vi "DrawPaticle.vi"(1 "Particle Measurements (Pixels) (左引脚)":dbl[][](array[numeric]), 2 "引用句柄输入":T1) -> (0 "Paticle中心数组":cluster{"Numeric":dbl, "Numeric":dbl}[](array[cluster]))   [LabVIEW 2014]
uses:
  <vilib>/vision/Image Controls.llb/IMAQ Image.ctl
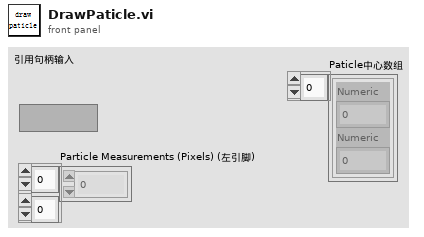
[diagram p1: front panel]
types:
  T1 = typedef "IMAQ Image.ctl" = refnum<image>
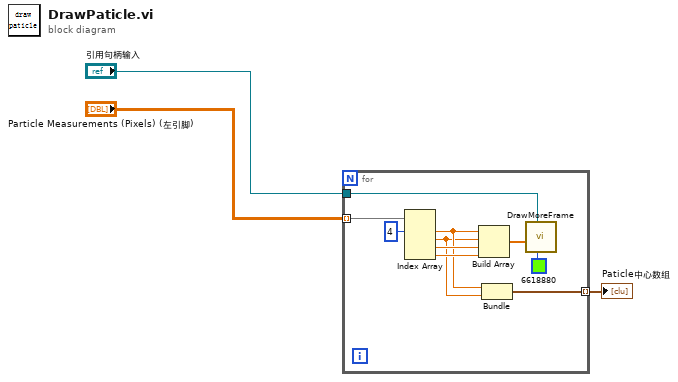
[diagram p0: block diagram]
diagram:
  n1 = for {
    tunnel: "Particle Measurements (Pixels) (左引脚)" -> [w13] mode=indexing
    tunnel: "引用句柄输入" -> [w9]
    tunnel: [w4] -> w1 mode=indexing
    n2 = Index Array(array=w13, index #1=4 ("索引")) -> (element #1=w6:dbl, element #2=w5:dbl, element #3=w12:dbl, element #4=w11:dbl)  [unwired: 3 in]
    n3 = Build Array(w6, w5, w12, w11) -> (w10:dbl[])
    n4 = Bundle("Numeric"=w6, "Numeric"=w5) -> (w4:cluster{"Numeric":dbl, "Numeric":dbl})  [unwired: 1 in]
    n5 = call "DrawMoreFrame.vi"("Color"=u32 6618880, "Image Out 2"=w9, "Rect_Center"=w10) -> ()  [unwired: 4 in, 1 out]
  }
  "Paticle中心数组" <- w1
